vi "Hide scrollbar.vi"(8 "error in (no error)":errorcluster, 11 "VI Refnum":refnum<vi>) -> (0 "error out":errorcluster)   [LabVIEW 2017, in "Toolbox.lvlib"]
uses:
  Toolbox.lvlib
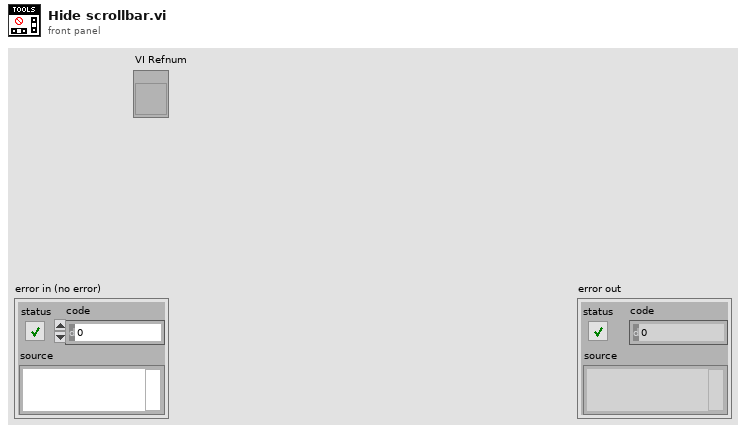
[diagram p1: front panel]
types:
  T1 = enum16{"Always On", "Always Off", "Off While Running"}
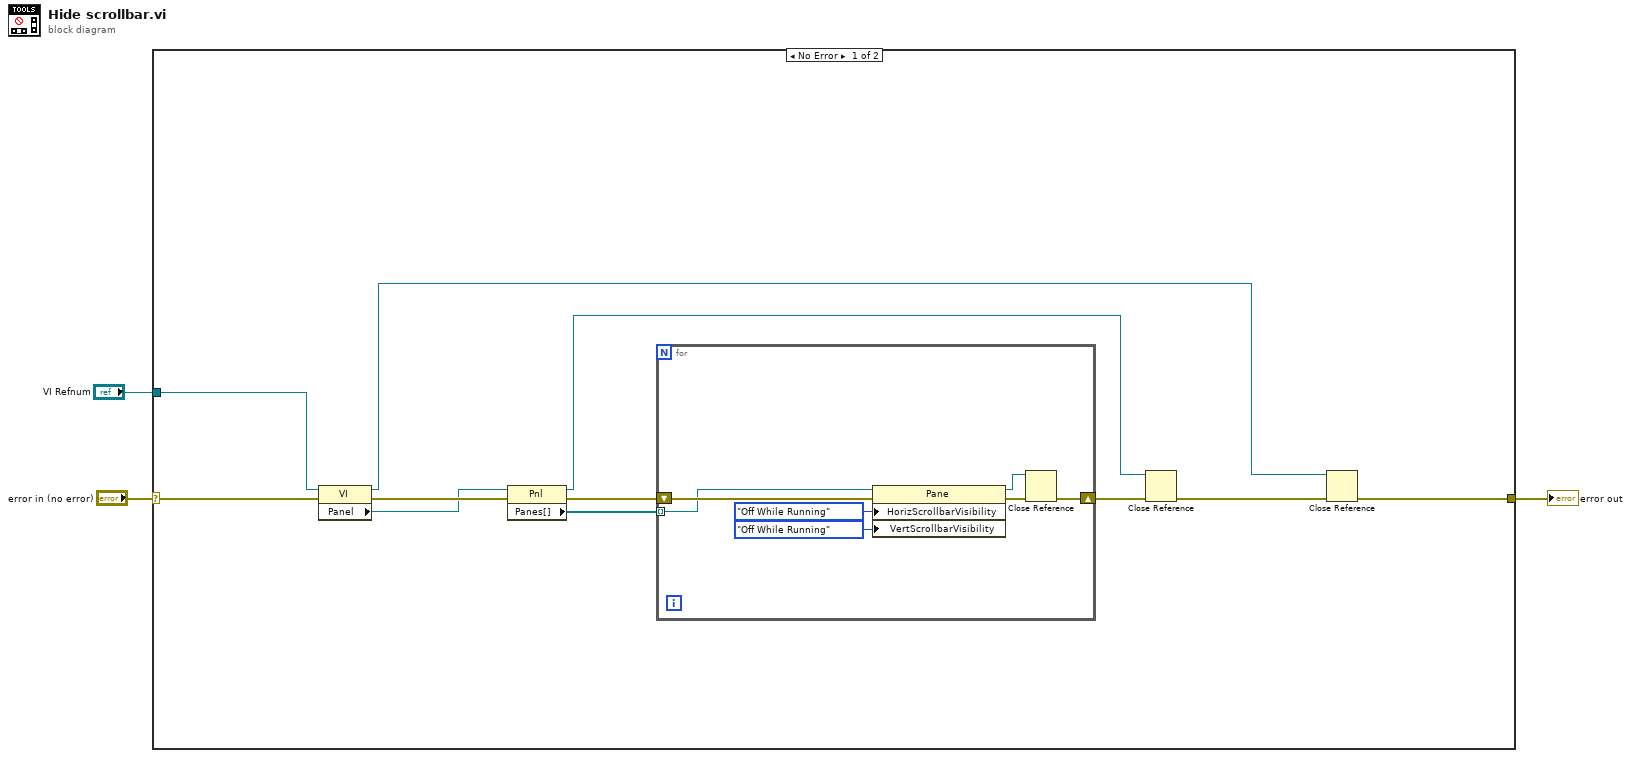
[diagram p0: block diagram]
diagram:
  n1 = case shown="No Error" "error in (no error)" {
    selector: "error in (no error)" -> [w14 w22]
    tunnel: [w5 w22] -> w2
    tunnel: "VI Refnum" -> [w11 _]
    frame No Error {
      n2 = property class="VI"(reference=w11, error in=w14) -> (reference out=w4:refnum<vi>, error out=w13:errorcluster, "Panel"=w10:refnum<vi>)
      n3 = property class="Pnl"(reference=w10, error in=w13) -> (reference out=w6:refnum<vi>, error out=w12:errorcluster, "Panes[]"=w8:refnum<vi>[])
      n4 = for {
        shift-right: [w16] -> w9
        shift-left: w12 -> [w21]
        tunnel: w8 -> [w19] mode=indexing
        n5 = property class="Pane"(reference=w19, error in=w21, "HorizScrollbarVisibility"=T1."Off While Running" ("Horizontal Scrollbar Visibility"), "VertScrollbarVisibility"=T1."Off While Running" ("Vertical Scrollbar Visibility")) -> (reference out=w15:refnum<vi>, error out=w20:errorcluster)
        n6 = Close Reference(reference=w15, error in (no error)=w20) -> (error out=w16:errorcluster)
      }
      n7 = Close Reference(reference=w6, error in (no error)=w9) -> (error out=w7:errorcluster)
      n8 = Close Reference(reference=w4, error in (no error)=w7) -> (error out=w5:errorcluster)
    }
    frame Error {
    }
  }
  "error out" <- w2
